vi "Blink Pass Fail Leds.vi"(7 "Sequence Context In":refnum<k7>, 8 "error in":errorcluster, 9 "Half Period (ms)":u32=100, 10 "Notification":string="TemperatureNotifier", 11 "Task In":refnum<k21>) -> (0 "error out":errorcluster)   [LabVIEW 2018]
uses:
  <vilib>/DAQmx/write.llb/DAQmx Write (Digital 1D Bool 1Chan 1Samp).vi
  <vilib>/DAQmx/miscellaneous.llb/DAQmx Fill In Error Info.vi
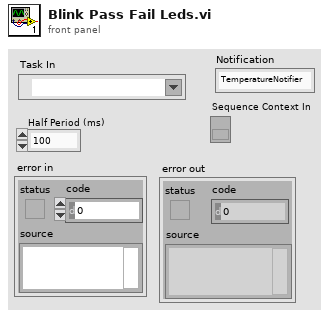
[diagram p1: front panel]
types:
  T1 = typedef "TestStand - Status Monitor.ctl" = cluster{"Sequence Context":refnum<k7>, "Execution":refnum<k7>, "Termination Monitor":refnum<k7>}
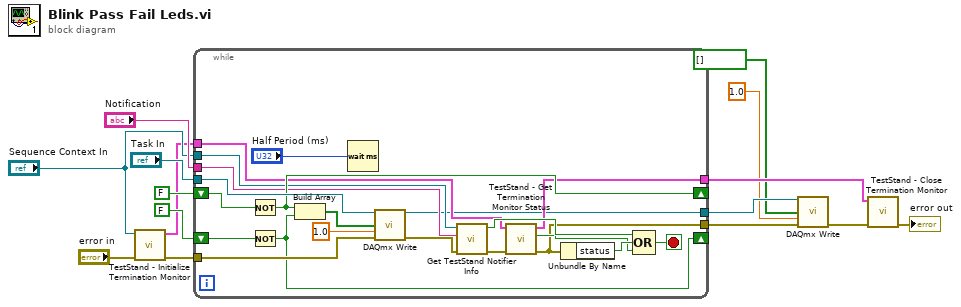
[diagram p0: block diagram]
diagram:
  n1 = call <vilib>:"TestStand - Initialize Termination Monitor.vi"("error in (no error)"="error in", "Sequence Context In"="Sequence Context In") -> ("error out"=w9:errorcluster, "Status Monitor Out"=w6:T1)  [unwired: 8 in]
  n2 = while {
    tunnel: "Task In" -> [w36]
    tunnel: w9 -> [w35]
    tunnel: [w19] -> w5
    shift-right: [w30] -> _
    shift-left: FALSE -> [w32]
    shift-right: [w29] -> _
    shift-left: FALSE -> [w31]
    tunnel: "Sequence Context In" -> [w27]
    tunnel: "Notification" -> [w25]
    tunnel: [w18] -> w10
    tunnel: w6 -> [w17]
    tunnel: [w16] -> w3
    stop <- w22 stop-if-true
    n3 = Not(x=w32) -> (.not. x?=w30:bool)
    n4 = Not(x=w31) -> (.not. x?=w29:bool)
    n5 = Build Array(w30, w29) -> (w33:bool[])
    n6 = Wait (ms)(milliseconds to wait="Half Period (ms)") -> ()  [unwired: 1 out]
    n7 = call-poly <vilib>:"DAQmx Write.vi"("task/channels in"=w36, "data"=w33, "timeout"=1.0, "error in"=w35) -> ("task out"=w16:refnum<k21>, "error out"=w26:errorcluster)  [unwired: 9 in, 1 out]
    n8 = call "Get TestStand Notifier Info.vi"("error in (no error)"=w26, "Notifier"=w25, "SequenceContext"=w27) -> ("error out"=w20:errorcluster, "Stop"=w24:bool)  [unwired: 7 in]
    n9 = call <vilib>:"TestStand - Get Termination Monitor Status.vi"("error in (no error)"=w20, "Status Monitor In"=w17) -> ("error out"=w19:errorcluster, "Terminating or Aborting"=w21:bool, "Status Monitor Out"=w18:T1)  [unwired: 7 in]
    n10 = Unbundle By Name(w19) -> ("status"=w23:bool)
    n11 = Compound Arithmetic op=OR(w24, w23, w21) -> (w22:bool)
  }
  n12 = call-poly <vilib>:"DAQmx Write.vi"("task/channels in"=w3, "data"=bool[] [], "timeout"=1.0, "error in"=w5) -> ("error out"=w4:errorcluster)  [unwired: 9 in, 2 out]
  n13 = call <vilib>:"TestStand - Close Termination Monitor.vi"("error in (no error)"=w4, "Status Monitor In"=w10) -> ("error out"=→"error out":errorcluster)  [unwired: 9 in]
